vi "Data Receiver.vi"() -> ()   [LabVIEW 2021]
panel:
  out "error out":errorcluster
  in  "error in":errorcluster
  in  "Pilot Address":string="localhost"
  out "Waveform Graph":dbl[](graph)
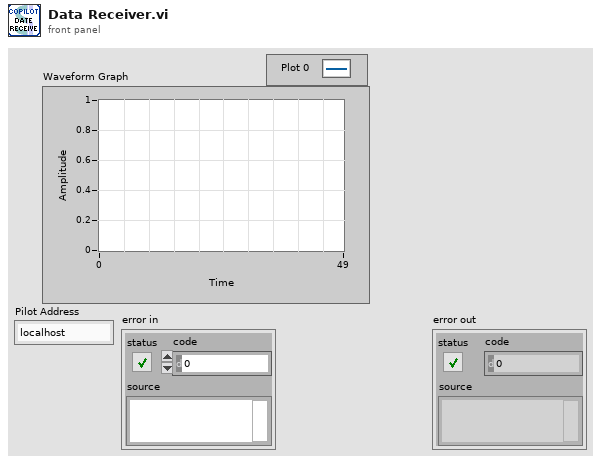
[diagram p1: front panel]
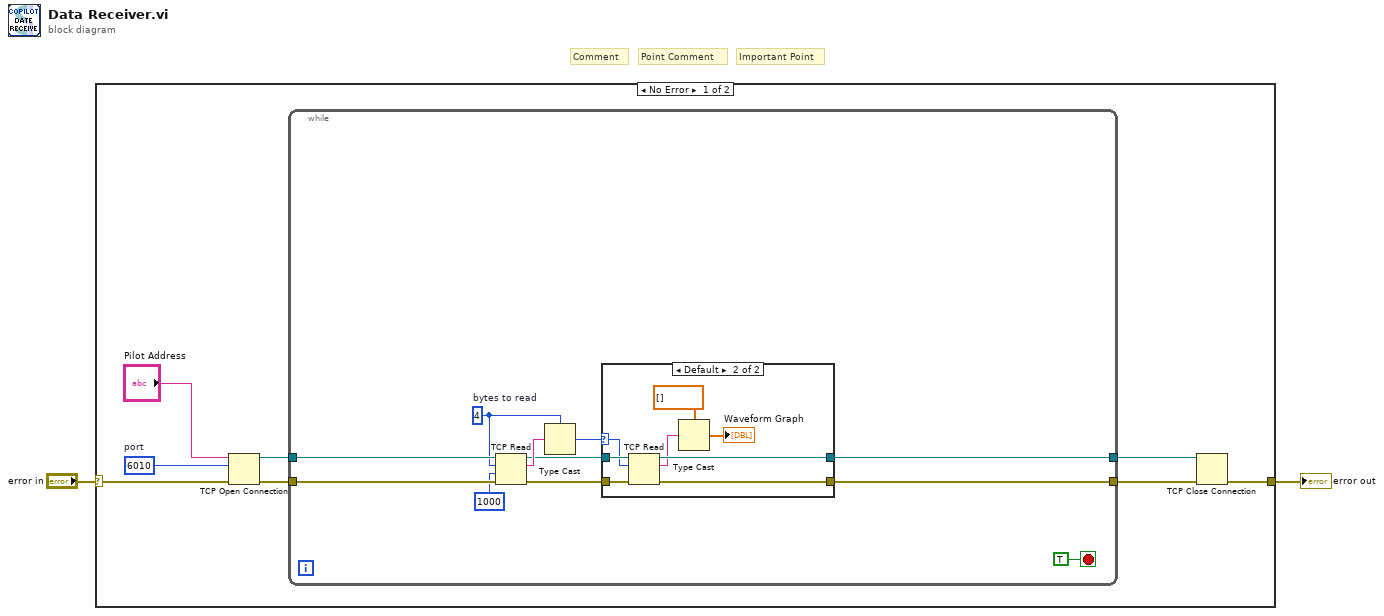
[diagram p0: block diagram]
diagram:
  # "Important Point"
  # "Point Comment"
  # "Comment"
  n1 = case shown="No Error" "error in" {
    selector: "error in" -> [w8 w32]
    tunnel: [w3 w32] -> w2
    frame No Error {
      w9 = u16 6010  # port
      n2 = TCP Open Connection(address="Pilot Address", remote port or service name=w9, error in (no error)=w8) -> (connection ID=w6:refnum<k5>, error out=w7:errorcluster)  [unwired: 2 in]
      n3 = while {
        tunnel: w7 -> [w19]
        tunnel: w6 -> [w20]
        tunnel: [w11] -> w5
        tunnel: [w12] -> w4
        stop <- TRUE stop-if-true
        w15 = 4  # bytes to read
        n4 = TCP Read(connection ID=w20, bytes to read=w15, error in (no error)=w19, 9:1000 ("timeout ms (25000)")) -> (connection ID out=w17:refnum<k5>, data out=w18:string, error out=w16:errorcluster)  [unwired: 1 in]
        n5 = Type Cast(type=w15, x=w18) -> (*(type *) &x=w14:i32)
        n6 = case shown="Default" w14 {
          selector: w14 -> [_ w24]
          tunnel: w17 -> [w23 w31]
          tunnel: w16 -> [w22 w30]
          tunnel: [w23 w27] -> w12
          tunnel: [w22 w26] -> w11
          frame ..0 {
            # "The server has not written any data"
          }
          frame Default {
            n7 = TCP Read(connection ID=w31, bytes to read=w24, error in (no error)=w30) -> (connection ID out=w27:refnum<k5>, data out=w25:string, error out=w26:errorcluster)  [unwired: 2 in]
            n8 = Type Cast(type=dbl[] [] ("chart"), x=w25) -> (*(type *) &x=→"Waveform Graph":dbl[])
          }
        }
      }
      n9 = TCP Close Connection(connection ID=w4, error in (no error)=w5) -> (error out=w3:errorcluster)  [unwired: 1 in, 1 out]
    }
    frame Error {
    }
  }
  "error out" <- w2
